vi "setChannelDefaults.vi"(8 "error in (no error)":errorcluster, 9 "Data":variant, 10 "physicalChannels":string[](array[string]), 11 "SpinCore in":refnum<class "SpinCore.lvclass">) -> (0 "error out":errorcluster, 3 "SpinCore out":refnum<class "SpinCore.lvclass">)   [LabVIEW 2009, in "Hardware.lvlib" / "Channels.lvlib" / "SpinCore.lvclass"]
doc: "Default Data Cluster:\n\n1) frequency (db)\n2) amplitude (db)\n3) phase (db)\n4) type (enum: sine, square, triangle)"
uses:
  SpinCore.lvclass
  Generic/DDSOutput.lvclass
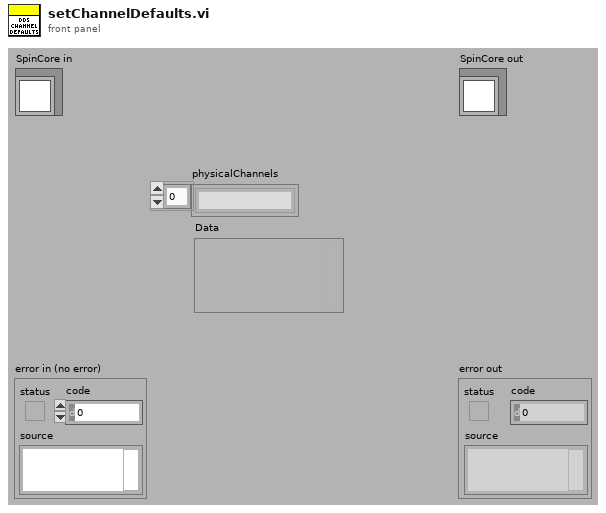
[diagram p1: front panel]
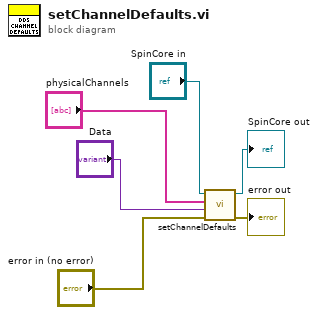
[diagram p0: block diagram]
diagram:
  n1 = call-parent "setChannelDefaults.vi"("error in (no error)"="error in (no error)", "Data"="Data", "physicalChannels"="physicalChannels", "DDSOutput in"="SpinCore in") -> ("error out"=→"error out":errorcluster, "DDSOutput out"=→"SpinCore out":refnum<class "SpinCore.lvclass">)  [unwired: 6 in]
